vi "MicroPulse - decode voltage.vi"(6 "start index":i32, 7 "voltage bytes":u8[](array[numeric])) -> (2 "volts read":dbl, 3 "voltage setting":dbl)   [LabVIEW 2026, in "MicroPulse_Driver.lvlib"]
uses:
  MicroPulse_Driver.lvlib
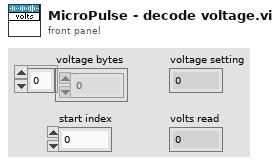
[diagram p1: front panel]
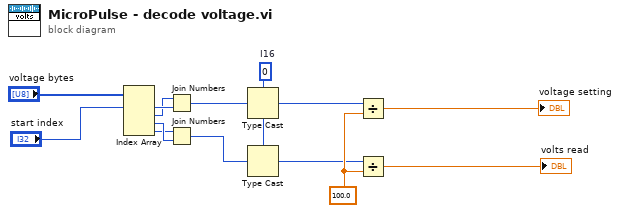
[diagram p0: block diagram]
diagram:
  w6 = i16 0  # I16
  w8 = 100.0 ("y")
  n1 = Index Array(array="voltage bytes", index #1="start index") -> (element #1=w12:u8, element #2=w11:u8, element #3=w10:u8, element #4=w9:u8)  [unwired: 3 in]
  n2 = Join Numbers(hi=w11, lo=w12) -> ((hi.lo)=w2:u16)
  n3 = Join Numbers(hi=w9, lo=w10) -> ((hi.lo)=w1:u16)
  n4 = Type Cast(type=w6, x=w2) -> (*(type *) &x=w7:i16)
  n5 = Type Cast(type=w6, x=w1) -> (*(type *) &x=w5:i16)
  n6 = Divide(x=w7, y=w8) -> (x/y=→"voltage setting":dbl)
  n7 = Divide(x=w5, y=w8) -> (x/y=→"volts read":dbl)
